vi "Initialize.vi"(8 "error in":errorcluster, 11 "UDP in":refnum<class "UDP.lvclass">) -> (0 "error out":errorcluster, 3 "UDP out":refnum<class "UDP.lvclass">)   [LabVIEW 2020, in "Plugin Instrument Driver.lvlib" / "UDP.lvclass"]
doc: "Creates an UDP Connection handled for the configured Port Number."
uses:
  UDP.lvclass
  Typedefs/Device Details.ctl
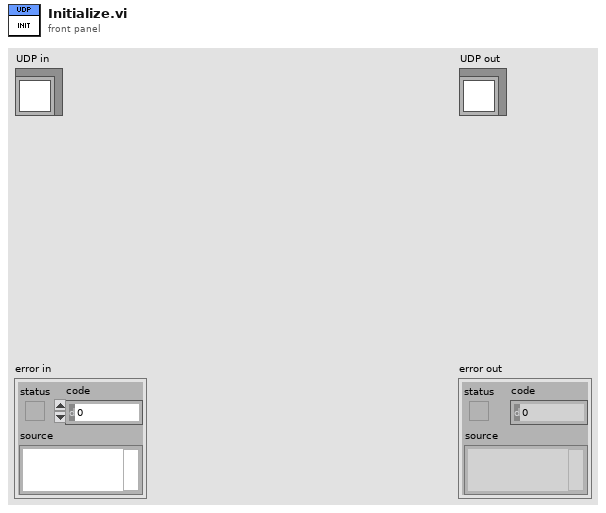
[diagram p1: front panel]
types:
  T1 = typedef "Plugin Instrument Driver.lvlib/UDP.lvclass/Device Details.ctl" = cluster{"Device Port Number":u16, "Device IP":string, "Timeout":i32, "Port Number":u16, "Connection ID":refnum<k16>}
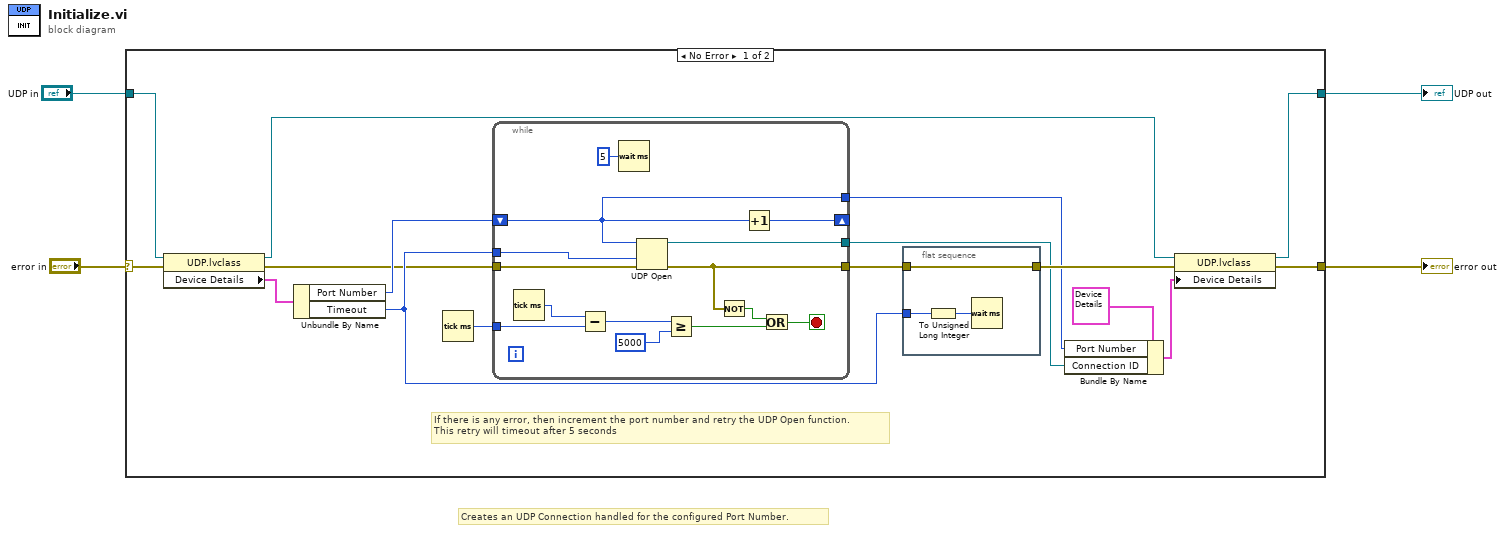
[diagram p0: block diagram]
diagram:
  # "Creates an UDP Connection handled for the configured Port Number."
  n1 = case shown="No Error" "error in" {
    selector: "error in" -> [w13 w38]
    tunnel: "UDP in" -> [w15 w39]
    tunnel: [w17 w38] -> w2
    tunnel: [w16 w39] -> w1
    frame No Error {
      # "If there is any error, then increment the port number and retry the UDP Open function.\nThis retry will timeout after 5 seconds"
      n2 = property class="UDP.lvclass"(reference=w15, error in=w13) -> (reference out=w12:refnum<class "UDP.lvclass">, error out=w9:errorcluster, "Device Details"=w14:T1)
      n3 = Unbundle By Name(w14) -> ("Port Number"=w11:u16, "Timeout"=w10:i32)
      n4 = Tick Count (ms)() -> (millisecond timer value=w20:u32)
      n5 = while {
        tunnel: w10 -> [w37]
        tunnel: [w36] -> w6
        shift-right: [w34] -> _
        shift-left: w11 -> [w32]
        tunnel: w9 -> [w24]
        tunnel: [w35] -> w19
        tunnel: [w32] -> w7
        tunnel: w20 -> [w31]
        stop <- w26 stop-if-true
        n6 = Tick Count (ms)() -> (millisecond timer value=w30:u32)
        n7 = Subtract(x=w30, y=w31) -> (x-y=w25:u32)
        n8 = Wait (ms)(milliseconds to wait=u32 5) -> ()  [unwired: 1 out]
        n9 = UDP Open(8:w24, 9:w37, 11:w32) -> (port=w36:refnum<k16>, 0:w35:errorcluster)  [unwired: 2 in, 1 out]
        n10 = Greater Or Equal?(x=w25, y=u32 5000) -> (x >= y?=w27:bool)
        n11 = Not(x=w35) -> (.not. x?=w28:bool)
        n12 = Increment(x=w32) -> (x+1=w34:u16)
        n13 = Or(x=w28, y=w27) -> (x .or. y?=w26:bool)
      }
      n14 = flat-sequence {
        tunnel: [w23] -> w18
        tunnel: w19 -> [w23]
        tunnel: w10 -> [w22]
        frame #0 {
          n15 = To Unsigned Long Integer(number=w22) -> (unsigned 32bit integer=w21:u32)
          n16 = Wait (ms)(milliseconds to wait=w21) -> ()  [unwired: 1 out]
        }
      }
      n17 = Bundle By Name(cluster=T1 {"Device Port Number"=2001, "Device IP"="192.168.1.1.100", "Timeout"=5000, "Port Number"=1234, "Connection ID"=refnum} ("Device Details"), "Port Number"=w7, "Connection ID"=w6) -> (w5:T1)
      n18 = property class="UDP.lvclass"(reference=w12, error in=w18, "Device Details"=w5) -> (reference out=w16:refnum<class "UDP.lvclass">, error out=w17:errorcluster)
    }
    frame Error {
    }
  }
  "error out" <- w2
  "UDP out" <- w1
